vi "wcsxy2sph.vi"(8 "Y":dbl, 9 "X":dbl, 11 "Astrometry":T1) -> (0 "lon":dbl format="%.6g", 1 "lat":dbl format="%.6g", 3 "Astrometry Dup":T1)   [LabVIEW 2019]
panel:
  out "atan2(y,x)":dbl
  out "phi":dbl
  out "theta":dbl
  out "r":dbl
  out "yy":dbl
  out "xx":dbl
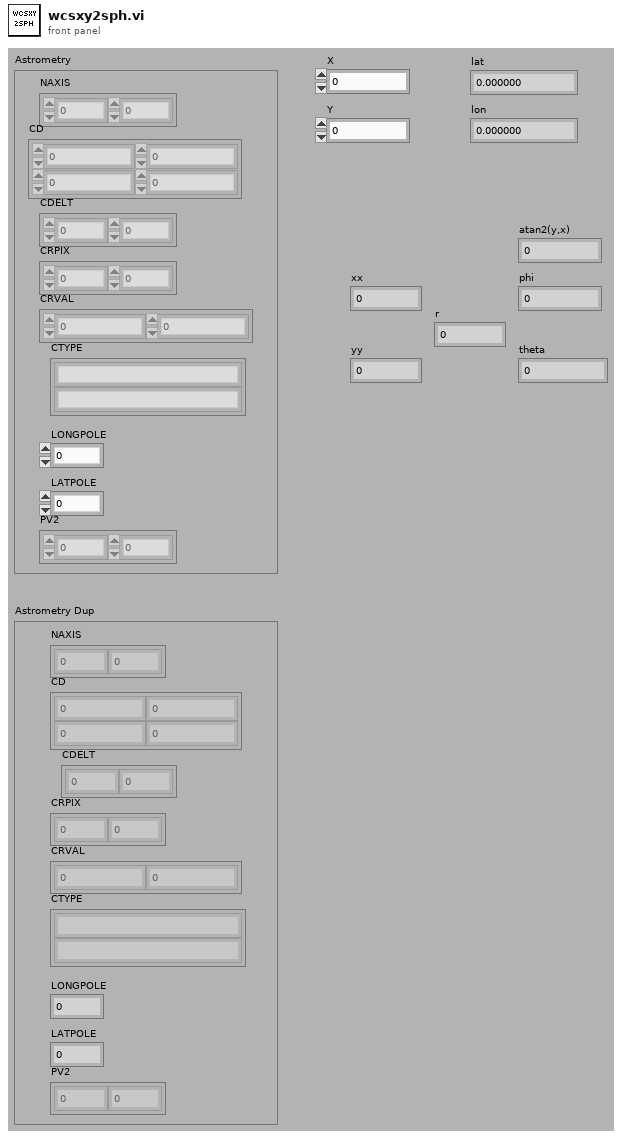
[diagram p1: front panel]
types:
  T1 = cluster{"NAXIS":dbl[], "CD":dbl[][], "CDELT":dbl[], "CRPIX":dbl[], "CTYPE":string[], "CRVAL":dbl[], "LONGPOLE":dbl, "LATPOLE":dbl, "PV2":dbl[]}
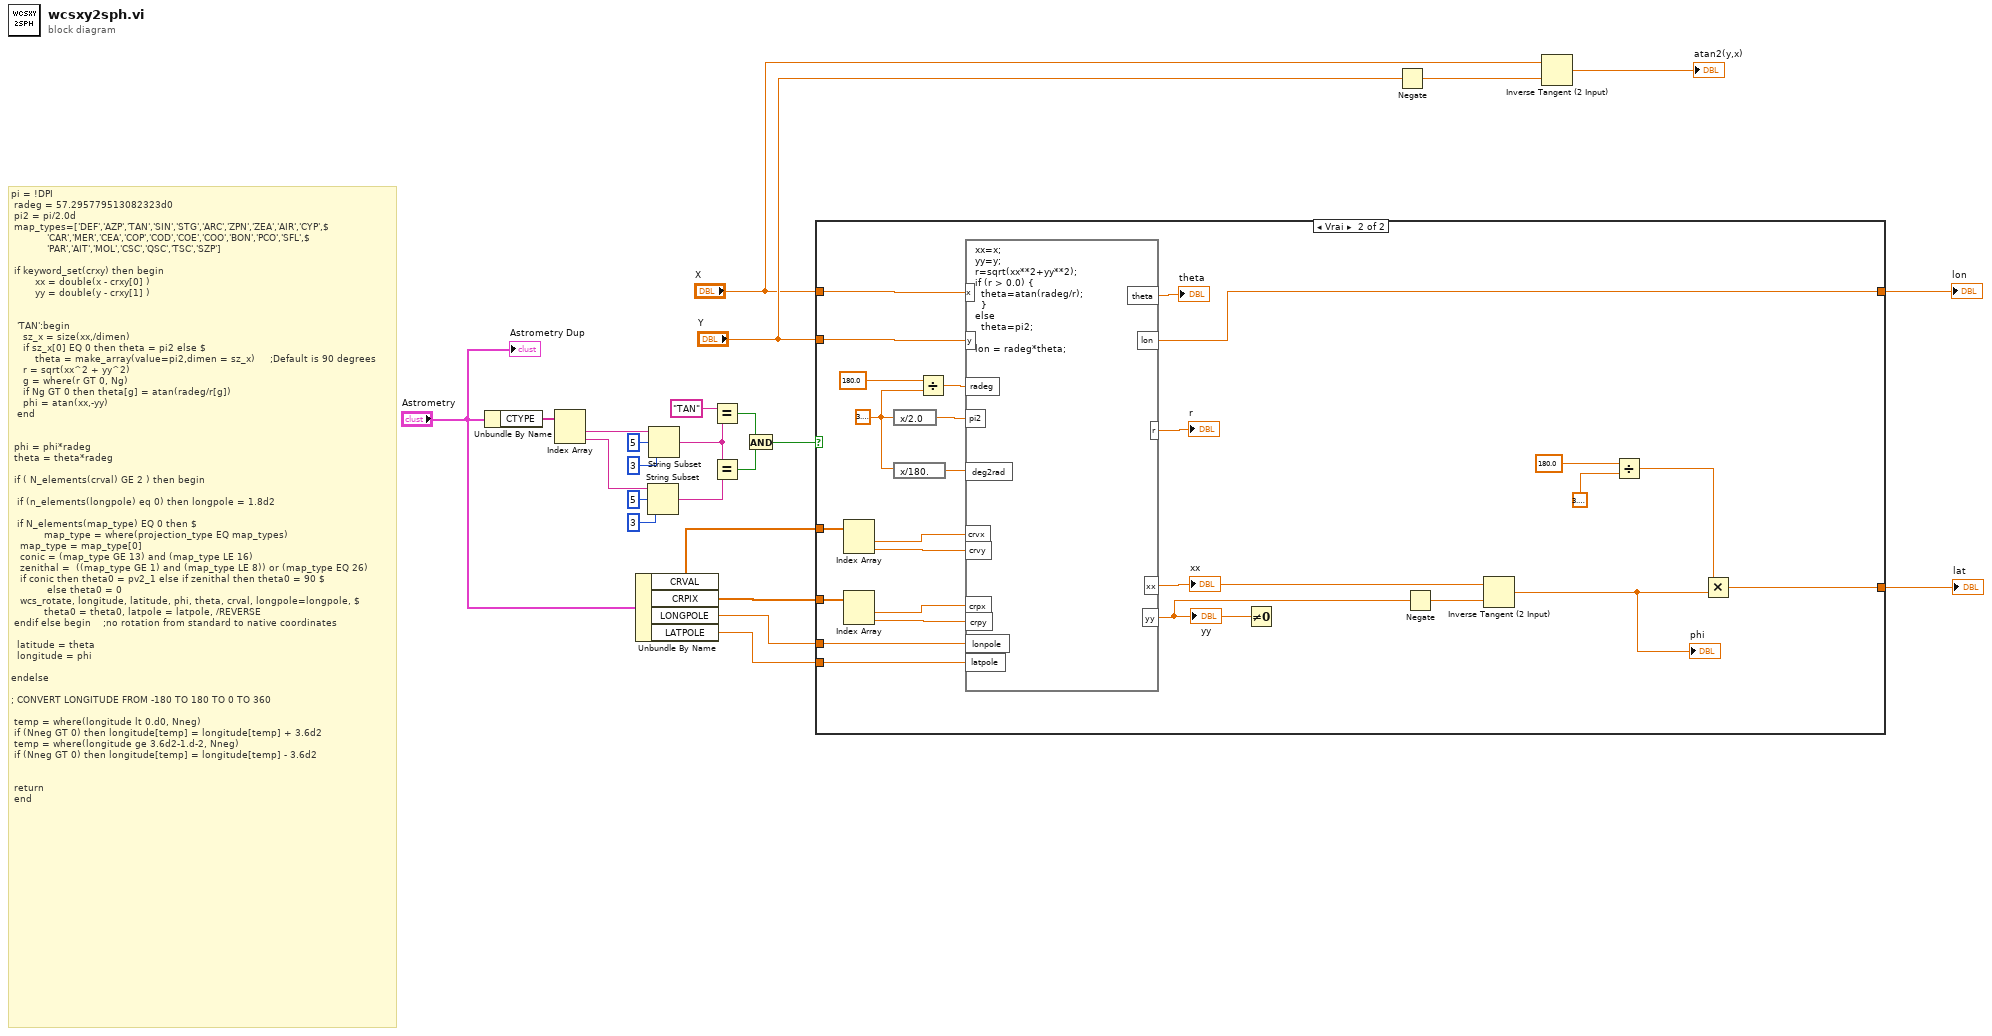
[diagram p0: block diagram]
diagram:
  # "pi = !DPI\n radeg = 57.295779513082323d0\n pi2 = pi/2.0d\n map_types=['DEF','AZP','TAN','SIN','STG','ARC','ZPN','ZEA','AIR','CYP',$\n            'CAR','MER','CEA','COP','COD','COE','COO','BON','PCO','SFL',$\n            'PAR','AIT','MOL','CSC','QSC','TSC','SZP']\n\n if keyword_set(crxy) then begin\n        xx = double(x - crxy[0] )\n        yy = double(y - crxy[1] )\n\n\n  'TAN':begin\n    sz_x = size(xx,/dimen)\n    if sz_x[0] EQ 0 then theta = pi2 else $\n        theta = make_array(value=pi2,dimen = sz_x)     ;Default is 90 degrees\n    r = sqrt(xx^2 + yy^2)\n    g = where(r GT 0, Ng)\n    if Ng GT 0 then theta[g] = atan(radeg/r[g]) \n    phi = atan(xx,-yy)\n  end\n\n\n phi = phi*radeg\n theta = theta*radeg\n \n if ( N_elements(crval) GE 2 ) then begin\n\n  if (n_elements(longpole) eq 0) then longpole = 1.8d2\n\n  if N_elements(map_type) EQ 0 then $\n           map_type = where(projection_type EQ map_types)\n   map_type = map_type[0]\n   conic = (map_type GE 13) and (map_type LE 16) \n   zenithal =  ((map_type GE 1) and (map_type LE 8)) or (map_type EQ 26) \n   if conic then theta0 = pv2_1 else if zenithal then theta0 = 90 $\n            else theta0 = 0 \n   wcs_rotate, longitude, latitude, phi, theta, crval, longpole=longpole, $\n           theta0 = theta0, latpole = latpole, /REVERSE\n endif else begin    ;no rotation from standard to native coordinates\n\n  latitude = theta\n  longitude = phi\n\nendelse\n\n; CONVERT LONGITUDE FROM -180 TO 180 TO 0 TO 360\n\n temp = where(longitude lt 0.d0, Nneg)\n if (Nneg GT 0) then longitude[temp] = longitude[temp] + 3.6d2\n temp = where(longitude ge 3.6d2-1.d-2, Nneg)\n if (Nneg GT 0) then longitude[temp] = longitude[temp] - 3.6d2\n\n\n return\n end"
  n1 = Unbundle By Name("Astrometry") -> ("CTYPE"=w24:string[])
  n2 = Index Array(array=w24) -> (element #1=w19:string, element #2=w18:string)  [unwired: 2 in]
  n3 = Unbundle By Name("Astrometry") -> ("CRVAL"=w10:dbl[], "CRPIX"=w11:dbl[], "LONGPOLE"=w9:dbl, "LATPOLE"=w8:dbl)
  n4 = String Subset(string=w18, offset (0)=5, length (rest)=3 ("length (rest)")) -> (substring=w17:string)
  n5 = String Subset(string=w19, offset (0)=5, length (rest)=3 ("length (rest)")) -> (substring=w16:string)
  n6 = Equal?(x="TAN", y=w16) -> (x = y?=w15:bool)
  n7 = Equal?(x=w16, y=w17) -> (x = y?=w14:bool)
  n8 = And(x=w15, y=w14) -> (x .and. y?=w12:bool)
  n9 = case shown="Vrai" w12 {
    tunnel: "X" -> [w25 w49]
    tunnel: "Y" -> [w26 w48]
    tunnel: w11 -> [_ w52]
    tunnel: w10 -> [_ w47]
    tunnel: w9 -> [_ w39]
    tunnel: w8 -> [_ w38]
    tunnel: [w26 w33] -> w2
    tunnel: [w25 w28] -> w1
    frame False {
    }
    frame True {
      w41 = 3.141592653589793
      n10 = Index Array(array=w47) -> (element #1=w45:dbl, element #2=w46:dbl)  [unwired: 2 in]
      n11 = Index Array(array=w52) -> (element #1=w51:dbl, element #2=w50:dbl)  [unwired: 2 in]
      n12 = expression code="x/2.0"(w41) -> (w44:dbl)
      n13 = expression code="x/180."(w41) -> (w40:dbl)
      n14 = Divide(x=180.0, y=w41) -> (x/y=w43:dbl)
      n15 = formula code="xx=x;\nyy=y;\nr=sqrt(xx**2+yy**2);\nif (r > 0.0) {\n  theta=atan(radeg/r);\n  }\nelse\n  theta=pi2;\n\nlon = radeg*theta;"("crpx"=w51, "crpy"=w50, "crvx"=w45, "crvy"=w46, "x"=w49, "y"=w48, "radeg"=w43, "pi2"=w44, "deg2rad"=w40, "latpole"=w38, "lonpole"=w39) -> ("lon"=w28:dbl, "xx"=w37:dbl, "yy"=w36:dbl, "r"=→"r":dbl, "theta"=→"theta":dbl)
      "xx" <- w37
      "yy" <- w36
      n16 = Not Equal To 0?(x=w36) -> ()  [unwired: 1 out]
      n17 = Negate(x=w36) -> (-x=w27:dbl)
      n18 = Inverse Tangent (2 Input)(1:w27, 2:w37) -> (0:w29:dbl)
      "phi" <- w29
      n19 = Divide(x=180.0, y=3.141592653589793) -> (x/y=w31:dbl)
      n20 = Multiply(x=w31, y=w29) -> (x*y=w33:dbl)
    }
  }
  "lat" <- w2
  "lon" <- w1
  n21 = Negate(x="Y") -> (-x=w4:dbl)
  n22 = Inverse Tangent (2 Input)(1:w4, 2:"X") -> (0:→"atan2(y,x)":dbl)
  "Astrometry Dup" <- "Astrometry"
